vi "Maui.Test.DefaultDirectory.WritePanelData.vi"(8 "error in (no error)":errorcluster, 11 "Maui.Test.DefaultDirectory in":refnum<class "Maui.Test.DefaultDirectory.lvclass">) -> (0 "error out":errorcluster, 3 "Maui.Test.DefaultDirectory out":refnum<class "Maui.Test.DefaultDirectory.lvclass">)   [LabVIEW 2020, in "Maui.Test.DefaultDirectory.lvclass"]
uses:
  Maui.Test.DefaultDirectory.lvclass
  <vilib>/addons/_JKI Toolkits/Caraya/classes/Test/Test.lvclass
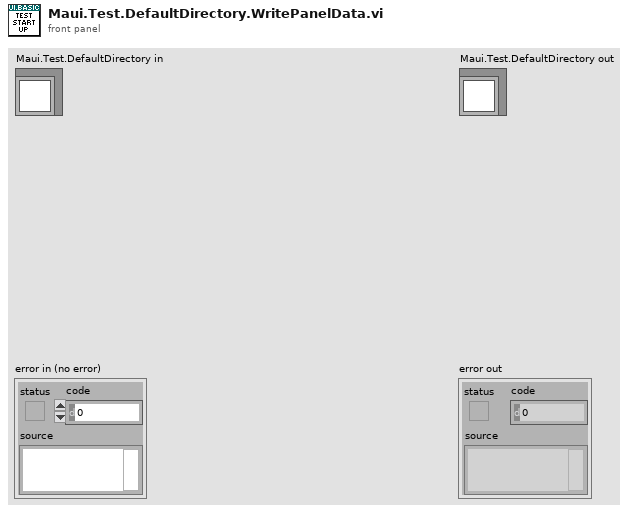
[diagram p1: front panel]
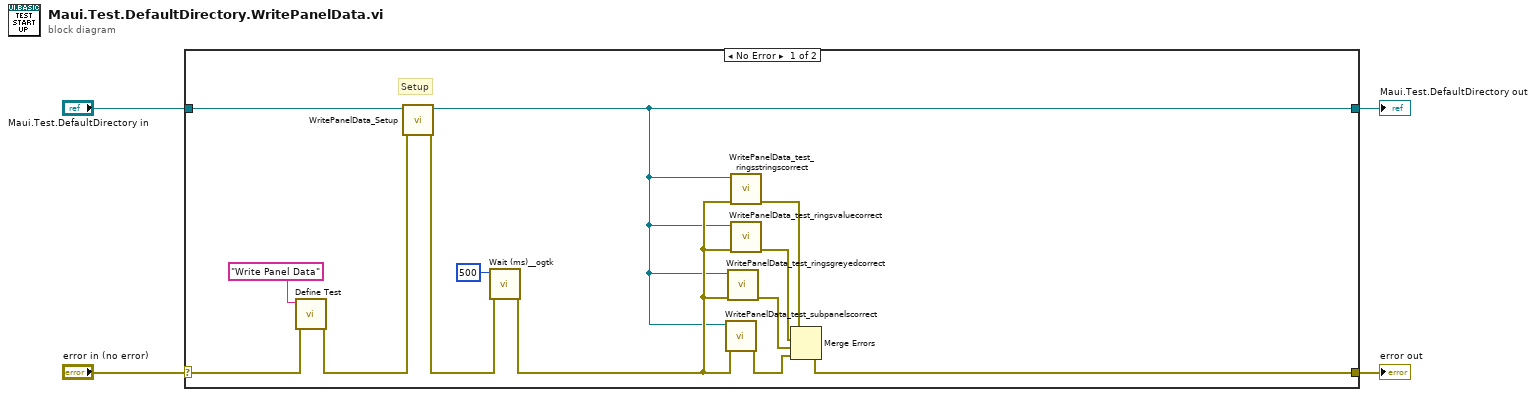
[diagram p0: block diagram]
diagram:
  n1 = case shown="No Error" "error in (no error)" {
    selector: "error in (no error)" -> [w16 w19]
    tunnel: [w9 w19] -> w3
    tunnel: [w6 w18] -> w1
    tunnel: "Maui.Test.DefaultDirectory in" -> [w14 w18]
    frame No Error {
      # "Setup"
      n2 = call <vilib>:"Define Test.vi"("error in (no error)"=w16, "Label (VI Title)"="Write Panel Data") -> ("error out"=w13:errorcluster)  [unwired: 9 in]
      n3 = call "WritePanelData_Setup.vi"("error in (no error)"=w13, "Maui.Test.DefaultDirectory in"=w14) -> ("error out"=w12:errorcluster, "Maui.Test.DefaultDirectory out"=w6:refnum<class "Maui.Test.DefaultDirectory.lvclass">)  [unwired: 8 in]
      n4 = call <userlib>:"Wait (ms)__ogtk.vi"("error in (no error)"=w12, "milliseconds to wait"=u32 500) -> ("error out"=w7:errorcluster)  [unwired: 8 in, 1 out]
      n5 = call "WritePanelData_test_subpanelscorrect.vi"("error in (no error)"=w7, "Maui.Test.DefaultDirectory in"=w6) -> ("error out"=w10:errorcluster)  [unwired: 8 in, 1 out]
      n6 = call "WritePanelData_test_ringsgreyedcorrect.vi"("error in (no error)"=w7, "Maui.Test.DefaultDirectory in"=w6) -> ("error out"=w11:errorcluster)  [unwired: 8 in, 1 out]
      n7 = call "WritePanelData_test_ringsstringscorrect.vi"("error in (no error)"=w7, "Maui.Test.DefaultDirectory in"=w6) -> ("error out"=w5:errorcluster)  [unwired: 8 in, 1 out]
      n8 = call "WritePanelData_test_ringsvaluecorrect.vi"("error in (no error)"=w7, "Maui.Test.DefaultDirectory in"=w6) -> ("error out"=w8:errorcluster)  [unwired: 8 in, 1 out]
      n9 = Merge Errors(w5, w8, w11, w10) -> (w9:errorcluster)
    }
    frame Error {
    }
  }
  "error out" <- w3
  "Maui.Test.DefaultDirectory out" <- w1
